vi "LeapYear.vi"(11 "Year":i32) -> (3 "Leap Year?":bool)   [LabVIEW 2015, in "Calendar.lvclass"]
uses:
  Calendar.lvclass
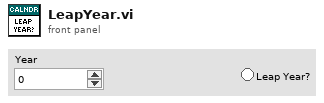
[diagram p1: front panel]
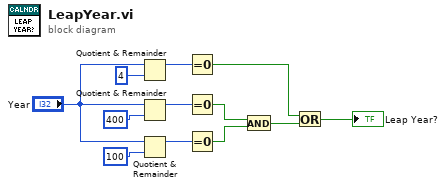
[diagram p0: block diagram]
diagram:
  n1 = Quotient & Remainder(x="Year", y=4) -> (x-y*floor(x/y)=w10:i32)  [unwired: 1 out]
  n2 = Quotient & Remainder(x="Year", y=400) -> (x-y*floor(x/y)=w5:i32)  [unwired: 1 out]
  n3 = Quotient & Remainder(x="Year", y=100) -> (x-y*floor(x/y)=w4:i32)  [unwired: 1 out]
  n4 = Equal To 0?(x=w10) -> (x = 0?=w9:bool)
  n5 = Equal To 0?(x=w5) -> (x = 0?=w2:bool)
  n6 = Equal To 0?(x=w4) -> (x = 0?=w3:bool)
  n7 = And(x=w2, y=w3) -> (x .and. y?=w1:bool)
  n8 = Or(x=w9, y=w1) -> (x .or. y?=→"Leap Year?":bool)
